vi "ERP_Graph.vi"() -> ()   [LabVIEW 2014]
uses:
  <vilib>/Analysis/baseanly.llb/Mean (DBL).vi
  <vilib>/Utility/file.llb/Read From Spreadsheet File (DBL).vi
  <vilib>/Utility/file.llb/Read From Spreadsheet File (I64).vi
  <vilib>/Analysis/NI_AALBase.lvlib
panel:
  out "Selected_Target":i32
  in  "selectedtarget.txt":path
  out "Icon6":dbl[][](graph)
  out "Icon5":dbl[][](graph)
  out "Icon4":dbl[][](graph)
  out "Icon3":dbl[][](graph)
  out "Icon2":dbl[][](graph)
  out "Icon1":dbl[][](graph)
  in  "Target_order.txtl":path
  in  "ERP_Total.txt":path
  in  "stop":bool
  out "Targer Number":i32
  in  "Trial_Number":i32=1
  # "(Emmerson et al, 1990)."
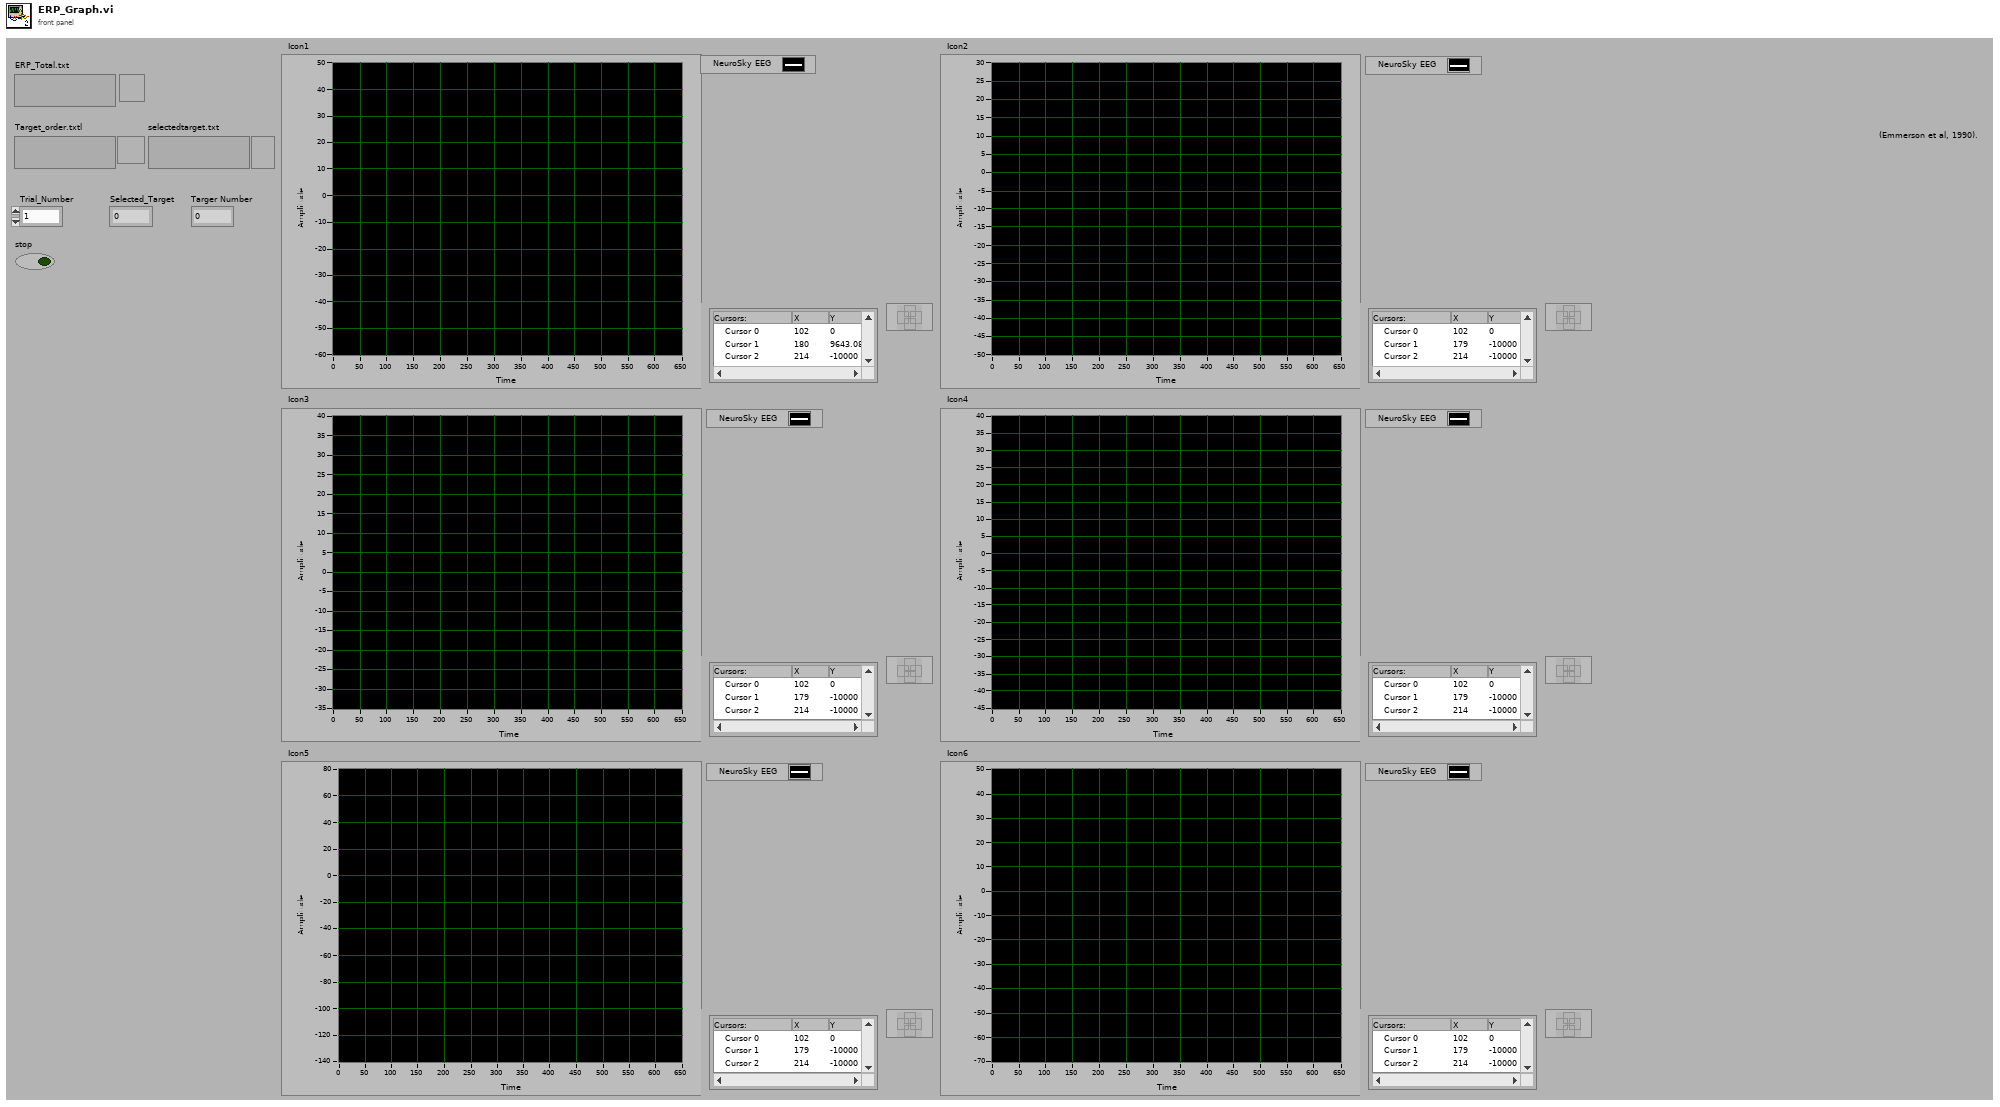
[diagram p1: front panel]
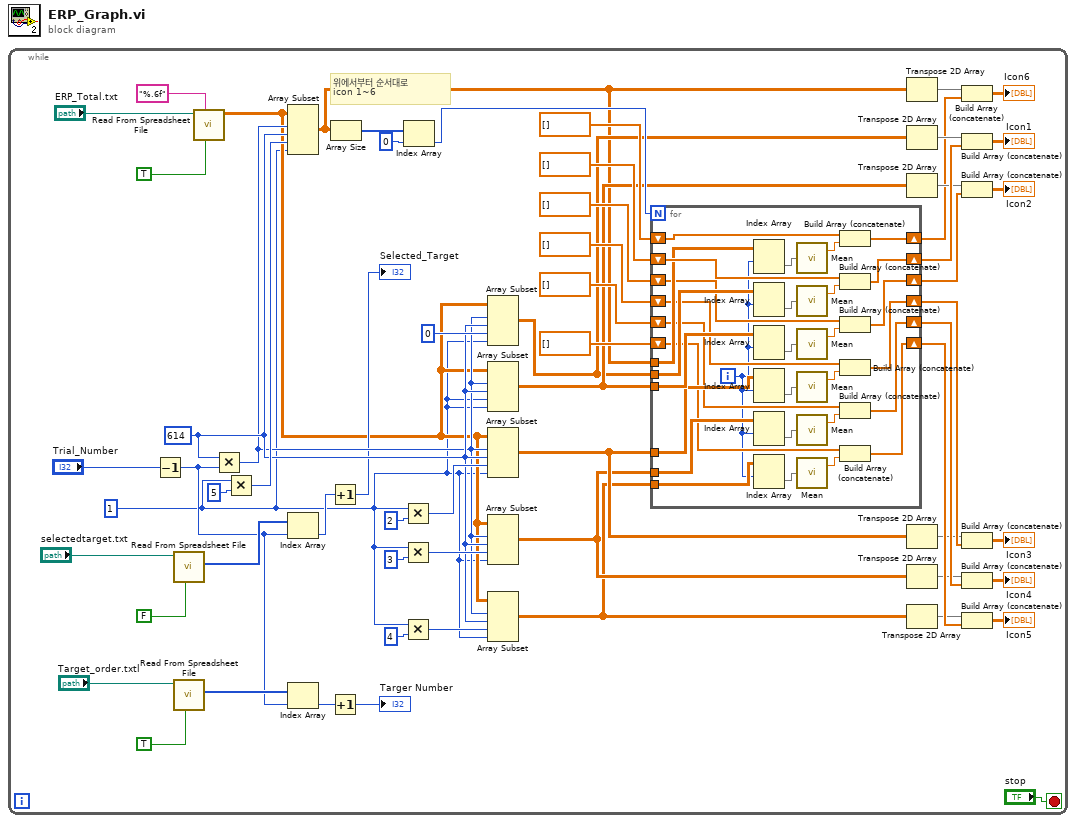
[diagram p0: block diagram]
diagram:
  n1 = while {
    stop <- "stop" stop-if-true
    w1 = 1 ("length")
    w51 = 614
    # "위에서부터 순서대로 \nicon 1~6"
    n2 = Decrement(x="Trial_Number") -> (x-1=w19:i32)
    n3 = call-poly <vilib>:"Read From Spreadsheet File.vi"("transpose (no:F)"=FALSE, "file path (dialog if empty)"="selectedtarget.txt") -> ("first row"=w21:i64[])  [unwired: 5 in, 4 out]
    n4 = call-poly <vilib>:"Read From Spreadsheet File.vi"("transpose (no:F)"=TRUE, "file path (dialog if empty)"="Target_order.txtl") -> ("first row"=w20:i64[])  [unwired: 5 in, 4 out]
    n5 = call-poly <vilib>:"Read From Spreadsheet File.vi"("transpose (no:F)"=TRUE, "format (%.3f)"="%.6f", "file path (dialog if empty)"="ERP_Total.txt") -> ("all rows"=w25:dbl[][])  [unwired: 4 in, 4 out]
    n6 = Multiply(x=w51, y=w19) -> (x*y=w50:i32)
    n7 = Multiply(x=w1, y=5) -> (x*y=w53:i32)
    n8 = Array Subset(array=w25, index (row)=w50, length (row)=w51, index (col)=w53, length (col)=w1) -> (w15:dbl[][])
    n9 = Index Array(array=w21, index=w19) -> (element=w18:i64)
    n10 = Index Array(array=w20, index=w19) -> (element=w17:i64)
    n11 = Increment(x=w18) -> (x+1=→"Selected_Target":i64)
    n12 = Increment(x=w17) -> (x+1=→"Targer Number":i64)
    n13 = Array Size(array=w15) -> (size(s)=w46:i32[])
    n14 = Multiply(x=w1, y=2) -> (x*y=w56:i32)
    n15 = Multiply(x=w1, y=3) -> (x*y=w55:i32)
    n16 = Multiply(x=w1, y=4) -> (x*y=w54:i32)
    n17 = Index Array(array=w46, index=0 ("인덱스")) -> (element=w45:i32)
    n18 = Array Subset(array=w25, index (row)=w50, length (row)=w51, index (col)=0 ("index"), length (col)=w1) -> (w16:dbl[][])
    n19 = Array Subset(array=w25, index (row)=w50, length (row)=w51, index (col)=w1, length (col)=w1) -> (w36:dbl[][])
    n20 = Array Subset(array=w25, index (row)=w50, length (row)=w51, index (col)=w56, length (col)=w1) -> (w34:dbl[][])
    n21 = Array Subset(array=w25, index (row)=w50, length (row)=w51, index (col)=w55, length (col)=w1) -> (w32:dbl[][])
    n22 = Array Subset(array=w25, index (row)=w50, length (row)=w51, index (col)=w54, length (col)=w1) -> (w30:dbl[][])
    n23 = for {
      N: w45 -> [_]
      shift-right: [w90] -> w37
      shift-left: dbl[] [] -> [w91]
      tunnel: w16 -> [w89]
      tunnel: w36 -> [w83]
      tunnel: w34 -> [w82]
      tunnel: w32 -> [w81]
      tunnel: w30 -> [w80]
      tunnel: w15 -> [w79]
      shift-right: [w77] -> w35
      shift-left: dbl[] [] -> [w76]
      shift-right: [w74] -> w33
      shift-left: dbl[] [] -> [w73]
      shift-right: [w71] -> w31
      shift-left: dbl[] [] -> [w70]
      shift-right: [w66] -> w29
      shift-left: dbl[] [] -> [w65]
      shift-right: [w67] -> w2
      shift-left: dbl[] [] -> [w64]
      i -> [w63]
      n24 = Index Array(array=w79, index (row)=w63) -> (element=w84:dbl[])  [unwired: 1 in]
      n25 = Index Array(array=w89, index (row)=w63) -> (element=w93:dbl[])  [unwired: 1 in]
      n26 = Index Array(array=w83, index (row)=w63) -> (element=w88:dbl[])  [unwired: 1 in]
      n27 = Index Array(array=w82, index (row)=w63) -> (element=w87:dbl[])  [unwired: 1 in]
      n28 = Index Array(array=w81, index (row)=w63) -> (element=w86:dbl[])  [unwired: 1 in]
      n29 = Index Array(array=w80, index (row)=w63) -> (element=w85:dbl[])  [unwired: 1 in]
      n30 = call-poly <vilib>:"Mean.vi"("X"=w84) -> ("mean"=w68:dbl)  [unwired: 1 out]
      n31 = call-poly <vilib>:"Mean.vi"("X"=w93) -> ("mean"=w92:dbl)  [unwired: 1 out]
      n32 = call-poly <vilib>:"Mean.vi"("X"=w88) -> ("mean"=w78:dbl)  [unwired: 1 out]
      n33 = call-poly <vilib>:"Mean.vi"("X"=w87) -> ("mean"=w75:dbl)  [unwired: 1 out]
      n34 = call-poly <vilib>:"Mean.vi"("X"=w86) -> ("mean"=w72:dbl)  [unwired: 1 out]
      n35 = call-poly <vilib>:"Mean.vi"("X"=w85) -> ("mean"=w69:dbl)  [unwired: 1 out]
      n36 = Build Array (concatenate)(w64, w68) -> (w67:dbl[])
      n37 = Build Array (concatenate)(w91, w92) -> (w90:dbl[])
      n38 = Build Array (concatenate)(w76, w78) -> (w77:dbl[])
      n39 = Build Array (concatenate)(w73, w75) -> (w74:dbl[])
      n40 = Build Array (concatenate)(w70, w72) -> (w71:dbl[])
      n41 = Build Array (concatenate)(w65, w69) -> (w66:dbl[])
    }
    n42 = Transpose 2D Array(2D array=w15) -> (transposed array=w9:dbl[][])
    n43 = Transpose 2D Array(2D array=w16) -> (transposed array=w14:dbl[][])
    n44 = Transpose 2D Array(2D array=w36) -> (transposed array=w13:dbl[][])
    n45 = Transpose 2D Array(2D array=w34) -> (transposed array=w12:dbl[][])
    n46 = Transpose 2D Array(2D array=w32) -> (transposed array=w11:dbl[][])
    n47 = Transpose 2D Array(2D array=w30) -> (transposed array=w10:dbl[][])
    n48 = Build Array (concatenate)(w9, w2) -> (→"Icon6":dbl[][])
    n49 = Build Array (concatenate)(w14, w37) -> (→"Icon1":dbl[][])
    n50 = Build Array (concatenate)(w13, w35) -> (→"Icon2":dbl[][])
    n51 = Build Array (concatenate)(w12, w33) -> (→"Icon3":dbl[][])
    n52 = Build Array (concatenate)(w11, w31) -> (→"Icon4":dbl[][])
    n53 = Build Array (concatenate)(w10, w29) -> (→"Icon5":dbl[][])
  }
